vi "Write dt.vi"(8 "error in (no error)":errorcluster, 10 "dt":dbl, 11 "Data1D in":refnum<class "Data1D.lvclass">) -> (0 "error out":errorcluster, 3 "Data1D out":refnum<class "Data1D.lvclass">)   [LabVIEW 2014, in "Data1D.lvclass"]
uses:
  Data1D.lvclass
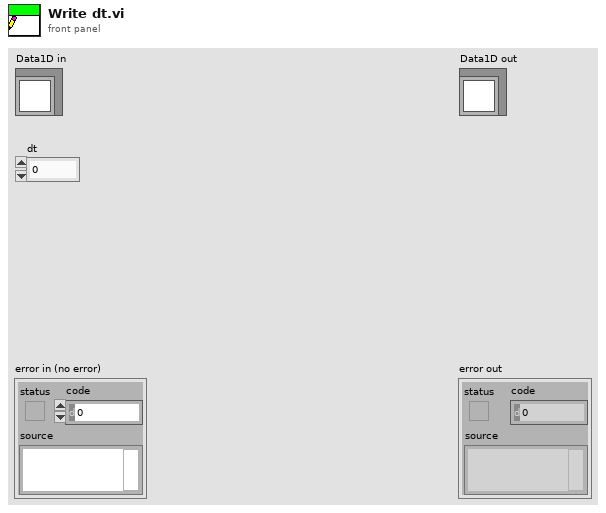
[diagram p1: front panel]
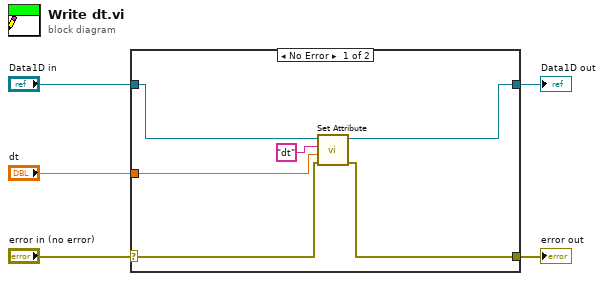
[diagram p0: block diagram]
diagram:
  n1 = case shown="No Error" "error in (no error)" {
    selector: "error in (no error)" -> [w7 w12]
    tunnel: [w6 w12] -> w4
    tunnel: [w10 w13] -> w2
    tunnel: "Data1D in" -> [w9 w13]
    tunnel: "dt" -> [w8 _]
    frame No Error {
      n2 = call-dynamic "Set Attribute.vi"("error in (no error)"=w7, "Value"=w8, "Name"="dt", "AbstractData in"=w9) -> ("error out"=w6:errorcluster, "AbstractData out"=w10:refnum<class "Data1D.lvclass">)  [unwired: 5 in, 1 out]
    }
    frame Error {
    }
  }
  "error out" <- w4
  "Data1D out" <- w2
